vi "interpolate xy graph to even grid.vi"(8 "error in (no error)":errorcluster, 10 "interp options":T1={"# samples (0=auto)"=0, "auto maxmin"=TRUE, "x"={"max"=0.0, "min"=0.0}, "method"=1, "X is monotonic"=FALSE} {"method" items=["nearest", "linear", "spline", "cubic Hermite", "Lagrange"]}, 11 "raw":T2(graph)) -> (0 "error out":errorcluster, 1 "interpolated":cluster{"xi used":dbl[], "yi":dbl[]}(graph), 2 "mean y":dbl format="%0.2f", 3 "raw+interpolated":cluster{"xi used":dbl[], "yi":dbl[]}[](graph), 4 "Dxi (spacing)":dbl)   [LabVIEW 2020]
uses:
  interpolate xy graph options.ctl
  NI_Gmath.lvlib
  NI_AALBase.lvlib
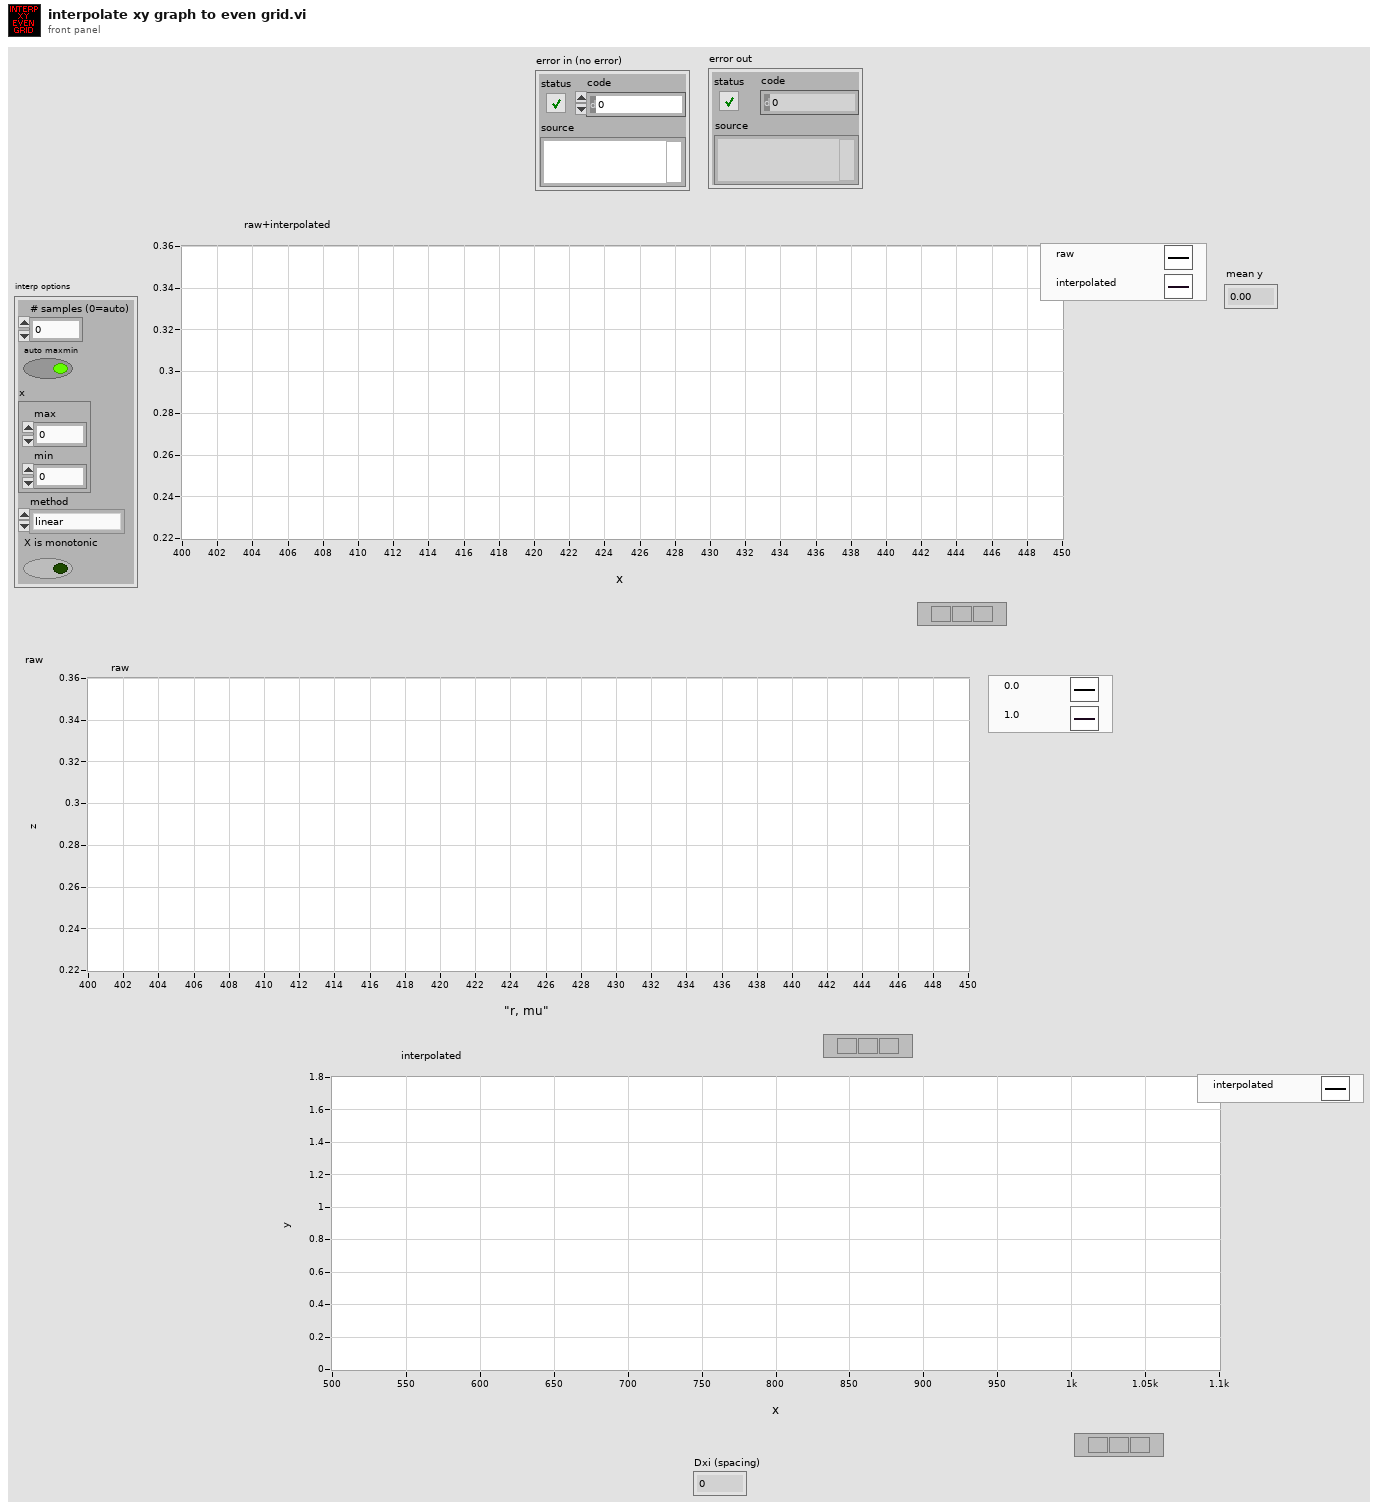
[diagram p1: front panel]
types:
  T1 = typedef "interpolate xy graph options.ctl" = cluster{"# samples (0=auto)":i32, "auto maxmin":bool, "x":cluster{"max":dbl, "min":dbl}, "method":i32, "X is monotonic":bool}
  T2 = cluster{"Sorted Array 2nd col out":dbl[], "3D data 1 scan line":dbl[]}
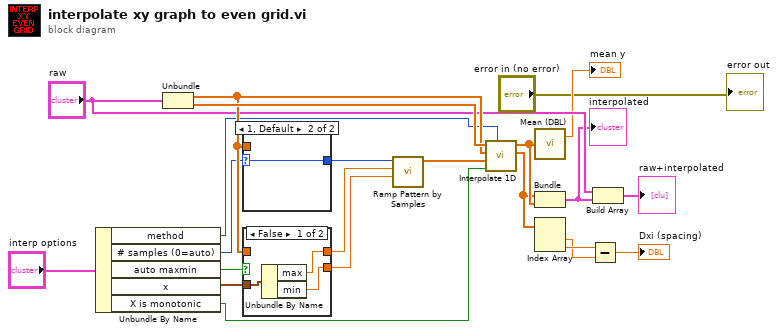
[diagram p0: block diagram]
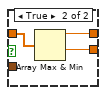
[diagram p2: hidden frame]
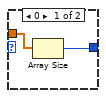
[diagram p3: hidden frame]
diagram:
  n1 = Unbundle By Name("interp options") -> ("method"=w3:i32, "# samples (0=auto)"=w6:i32, "auto maxmin"=w5:bool, "x"=w4:cluster{"max":dbl, "min":dbl}, "X is monotonic"=w2:bool)
  n2 = Unbundle("raw") -> ("Sorted Array 2nd col out"=w19:dbl[], "3D data 1 scan line"=w22:dbl[])
  n3 = case shown="1, Default" w6 {
    selector: w6 -> [_ w25]
    tunnel: w19 -> [w24 _]
    tunnel: [w23 w25] -> w18
    frame 0 {
      n4 = Array Size(array=w24) -> (size(s)=w23:i32)
    }
    frame 1, Default {
    }
  }
  n5 = case shown="False" w5 {
    tunnel: [w27 w31] -> w21
    tunnel: [w26 w30] -> w20
    tunnel: w19 -> [_ w29]
    tunnel: w4 -> [w28 _]
    frame False {
      n6 = Unbundle By Name(w28) -> ("max"=w27:dbl, "min"=w26:dbl)
    }
    frame True {
      n7 = Array Max & Min(array=w29) -> (max value=w31:dbl, min value=w30:dbl)  [unwired: 2 out]
    }
  }
  n8 = call "Ramp Pattern by Samples.vi"("start"=w20, "end"=w21, "samples"=w18) -> ("Ramp Pattern"=w17:dbl[])  [unwired: 7 in, 1 out]
  n9 = call "Interpolate 1D.vi"("method"=w3, "X is monotonic"=w2, "xi"=w17, "X"=w19, "Y"=w22) -> ("xi used"=w11:dbl[], "yi"=w14:dbl[])  [unwired: 4 in, 1 out]
  n10 = call "Mean (DBL).vi"("X"=w14) -> ("mean"=→"mean y":dbl)  [unwired: 1 out]
  n11 = Bundle("xi used"=w11, "yi"=w14) -> (w12:cluster{"xi used":dbl[], "yi":dbl[]})  [unwired: 1 in]
  "interpolated" <- w12
  n12 = Index Array(array=w11) -> (element #1=w9:dbl, element #2=w10:dbl)  [unwired: 2 in]
  n13 = Subtract(x=w10, y=w9) -> (x-y=→"Dxi (spacing)":dbl)
  n14 = Build Array("raw", w12) -> (→"raw+interpolated":cluster{"xi used":dbl[], "yi":dbl[]}[])
  "error out" <- "error in (no error)"
